vi "tcplink-server -- test.vi"() -> ()   [LabVIEW 2020]
uses:
  publisher action.ctl
  sparkle.ctl
panel:
  in  "millisecond multiple":u32=100
  in  "Stop":bool
  out "Gamma":dbl
  out "frequency":dbl
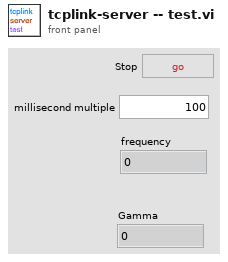
[diagram p1: front panel]
types:
  T1 = typedef "sparkle.ctl" = cluster{"units":string, "data":dbl}
  T2 = typedef "publisher action.ctl" = enum16{"set", "get", "init", "check"}
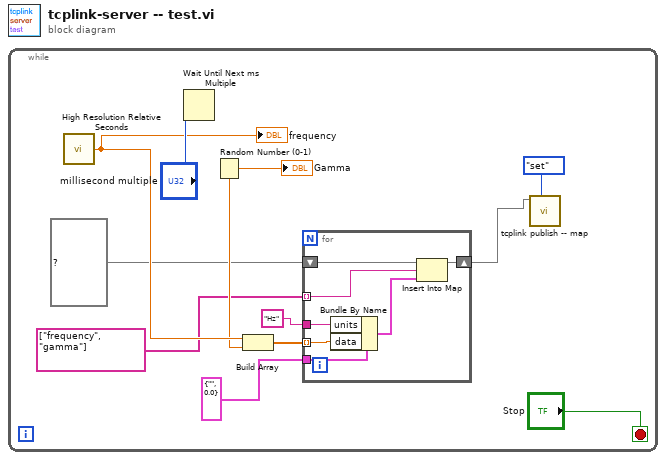
[diagram p0: block diagram]
diagram:
  n1 = while {
    stop <- "Stop" stop-if-true
    n2 = call <vilib>:"High Resolution Relative Seconds.vi"() -> ("relative seconds"=w8:dbl)
    "frequency" <- w8
    n3 = Wait Until Next ms Multiple(millisecond multiple="millisecond multiple") -> ()  [unwired: 1 out]
    n4 = Random Number (0-1)() -> (number: 0 to 1=w7:dbl)
    "Gamma" <- w7
    n5 = Build Array(w8, w7) -> (w3:dbl[])
    n6 = for {
      tunnel: string[] ["frequency", "gamma"] ("string array IN") -> [w18] mode=indexing
      shift-right: [w16] -> w4
      shift-left: map{string, T1} {} ("sparkle map IN") -> [w17]
      tunnel: w3 -> [w14] mode=indexing
      tunnel: T1 {"units"="", "data"=0.0} ("sparkle") -> [w15]
      tunnel: "Hz" ("units") -> [w12]
      n7 = Bundle By Name(cluster=w15, "units"=w12, "data"=w14) -> (w13:T1)
      n8 = Insert Into Map(map in=w17, key=w18, value=w13) -> (map out=w16:map{string, T1})  [unwired: 2 out]
    }
    n9 = call "tcplink publish -- map.vi"("publisher action"=publisher_action."set", "sparkle map IN"=w4) -> ()  [unwired: 9 in, 1 out]
  }
